vi "tcp rx.vi"(8 "error in":errorcluster, 9 "poll timeout ms (50)":i32=50, 10 "body rx timeout ms (5000)":i32=5000, 11 "TCP Connection in":refnum<k5>) -> (0 "error out":errorcluster, 1 "poll timeout":bool, 2 "rx":string, 3 "TCP Connection out":refnum<k5>)   [LabVIEW 2014]
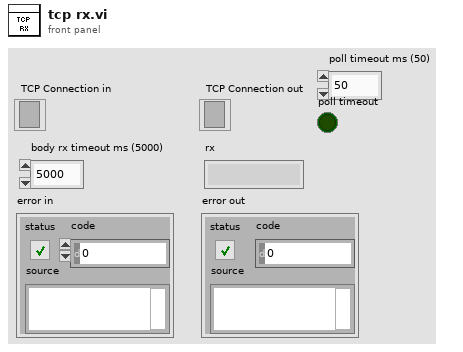
[diagram p1: front panel]
types:
  T1 = enum16{"Standard", "Buffered", "CRLF", "Immediate"}
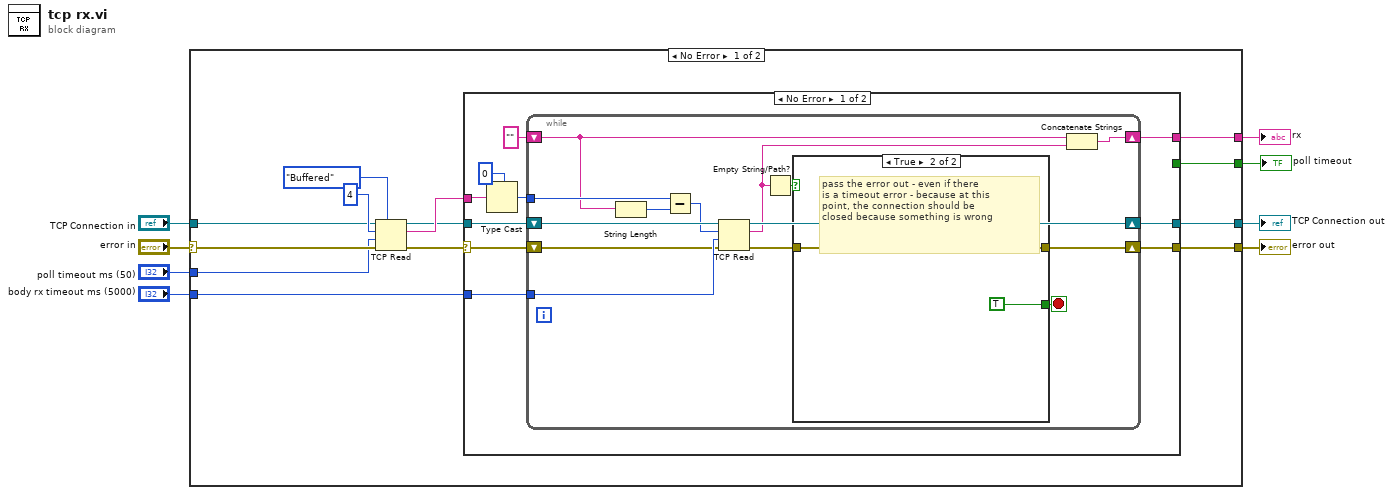
[diagram p0: block diagram]
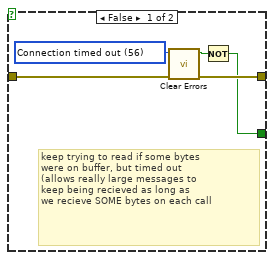
[diagram p2: hidden frame]
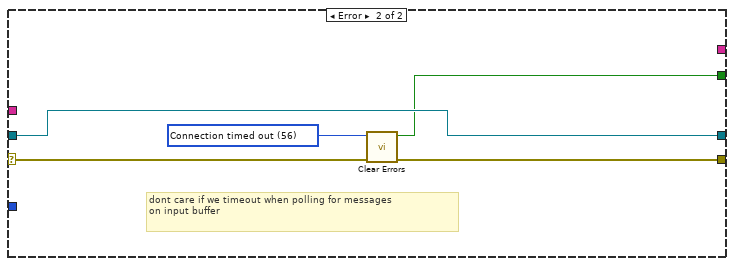
[diagram p3: hidden frame]
diagram:
  n1 = case shown="No Error" "error in" {
    selector: "error in" -> [w13 w58]
    tunnel: [w21 _] -> w8
    tunnel: [w20 w58] -> w7
    tunnel: [w19 w59] -> w6
    tunnel: "body rx timeout ms (5000)" -> [w18 _]
    tunnel: "TCP Connection in" -> [w14 w59]
    tunnel: "poll timeout ms (50)" -> [w11 _]
    tunnel: [w9 _] -> w1
    frame No Error {
      n2 = TCP Read(connection ID=w14, bytes to read=4, error in (no error)=w13, 7:T1."Buffered" ("mode (standard)"), 9:w11) -> (connection ID out=w16:refnum<k5>, data out=w17:string, error out=w10:errorcluster)
      n3 = case shown="No Error" w10 {
        selector: w10 -> [w26 w56]
        tunnel: [w31 _] -> w21
        tunnel: [w30 w55] -> w20
        tunnel: [w29 w57] -> w19
        tunnel: w18 -> [w28 _]
        tunnel: w17 -> [w23 _]
        tunnel: w16 -> [w27 w57]
        tunnel: [_ w53] -> w9
        frame No Error {
          n4 = Type Cast(type=0 ("length"), x=w23) -> (*(type *) &x=w22:i32)
          n5 = while {
            tunnel: w28 -> [w44]
            tunnel: w22 -> [w35]
            shift-right: [w45] -> w29
            shift-left: w27 -> [w43]
            shift-right: [w38] -> w30
            shift-left: w26 -> [w42]
            shift-right: [w41] -> w31
            shift-left: "" ("data out") -> [w33]
            stop <- w36 stop-if-true
            n6 = String Length(string=w33) -> (length=w32:i32)
            n7 = Subtract(x=w35, y=w32) -> (x-y=w34:i32)
            n8 = TCP Read(connection ID=w43, bytes to read=w34, error in (no error)=w42, 9:w44) -> (connection ID out=w45:refnum<k5>, data out=w40:string, error out=w37:errorcluster)  [unwired: 1 in]
            n9 = Empty String/Path?(string/path=w40) -> (empty?=w39:bool)
            n10 = case shown="True" w39 {
              tunnel: [w48 w52] -> w38
              tunnel: w37 -> [w49 w52]
              tunnel: [w46 TRUE] -> w36
              frame False {
                w50 = 56 items=["No Error", "Argument Error", "Memory Full", "Out of Zone", "End of File", "File Already Open", "Generic File IO Error", "File Not Found", "File Permission Error", "Disk Full", "Duplicate Path", "Too Many Files Open", "Not Enabled", "Resource File Not Found", "Cannot Add Resource", "Resource Not Found", "Image Not Found", "Image Memory Error", "Pen Does Not Exist", "Config Bad Type", "Config Token Not Found", "Config Parse Error", "Config Memory Error", "Bad External Code Format", "Bad External Code Offset", "External Code Not Present", "Null Window", "Destroy Window Mixup", "Null Menu", "Print Aborted", "Bad Print Record", "Print Driver Error", "Windows Error During Print", "Memory Error During Print", "Print Dialog Error", "Generic Print Error", "Invalid Device Refnum", "Device Not Found", "Device Parameter Error", "Device Unit Error", "Can't Open Device", "Device Call Aborted", "Generic Error", "Cancelled By User", "Object ID Too Low", "Object ID Too High", "Object Not In Heap", "Unknown Heap", "Bad DefProc ID", "DefProc Not In Table", "Message Out Of Range", "Null Method", "Unknown Message", "Manager Call Not Supported", "Bad address", "Connection In progress", "Connection timed out", "Connection is already in progress", "Network attribute not supported", "Network error", "Address in use", "System out of memory", "Connection aborted", "Connection refused", "Connection is not connected", "Connection is already connected", "Connection closed", "Initialize error (interapplication manager)", "Bad occurrence", "Wait on unbound occurrence handler", "Occurrence queue overflow", "Bad path", "Semaphore not signaled", "Unrecognized type (interapplication manager)"] ("1st Error to Convert")
                # "keep trying to read if some bytes\nwere on buffer, but timed out\n(allows really large messages to\nkeep being recieved as long as\nwe recieve SOME bytes on each call"
                n11 = call <vilib>:"Clear Errors.vi"("error in (no error)"=w49, "specific error code to clear (0: all)"=w50) -> ("error out"=w48:errorcluster, "specific error cleared?"=w47:bool)  [unwired: 4 in]
                n12 = Not(x=w47) -> (.not. x?=w46:bool)
              }
              frame True {
                # "pass the error out - even if there\nis a timeout error - because at this\npoint, the connection should be \nclosed because something is wrong"
              }
            }
            n13 = Concatenate Strings(w33, w40) -> (w41:string)
          }
        }
        frame Error {
          w54 = 56 items=["No Error", "Argument Error", "Memory Full", "Out of Zone", "End of File", "File Already Open", "Generic File IO Error", "File Not Found", "File Permission Error", "Disk Full", "Duplicate Path", "Too Many Files Open", "Not Enabled", "Resource File Not Found", "Cannot Add Resource", "Resource Not Found", "Image Not Found", "Image Memory Error", "Pen Does Not Exist", "Config Bad Type", "Config Token Not Found", "Config Parse Error", "Config Memory Error", "Bad External Code Format", "Bad External Code Offset", "External Code Not Present", "Null Window", "Destroy Window Mixup", "Null Menu", "Print Aborted", "Bad Print Record", "Print Driver Error", "Windows Error During Print", "Memory Error During Print", "Print Dialog Error", "Generic Print Error", "Invalid Device Refnum", "Device Not Found", "Device Parameter Error", "Device Unit Error", "Can't Open Device", "Device Call Aborted", "Generic Error", "Cancelled By User", "Object ID Too Low", "Object ID Too High", "Object Not In Heap", "Unknown Heap", "Bad DefProc ID", "DefProc Not In Table", "Message Out Of Range", "Null Method", "Unknown Message", "Manager Call Not Supported", "Bad address", "Connection In progress", "Connection timed out", "Connection is already in progress", "Network attribute not supported", "Network error", "Address in use", "System out of memory", "Connection aborted", "Connection refused", "Connection is not connected", "Connection is already connected", "Connection closed", "Initialize error (interapplication manager)", "Bad occurrence", "Wait on unbound occurrence handler", "Occurrence queue overflow", "Bad path", "Semaphore not signaled", "Unrecognized type (interapplication manager)"] ("1st Error to Convert")
          # "dont care if we timeout when polling for messages\non input buffer"
          n14 = call <vilib>:"Clear Errors.vi"("error in (no error)"=w56, "specific error code to clear (0: all)"=w54) -> ("error out"=w55:errorcluster, "specific error cleared?"=w53:bool)  [unwired: 4 in]
        }
      }
    }
    frame Error {
    }
  }
  "rx" <- w8
  "error out" <- w7
  "TCP Connection out" <- w6
  "poll timeout" <- w1
